vi "SmartSEM Remote API get float.vi"(8 "error in":errorcluster, 10 "lpszParam":string, 11 "ActiveX Container":refnum<k7>(container)) -> (0 "error out":errorcluster, 2 "vValue":sgl, 3 "reference out":refnum<k7>)   [LabVIEW 2018]
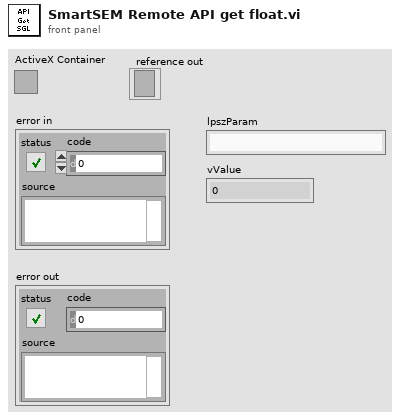
[diagram p1: front panel]
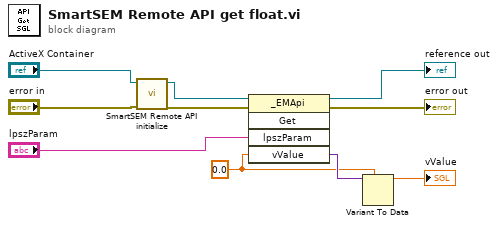
[diagram p0: block diagram]
diagram:
  w6 = sgl 0.0 ("vValue")
  n1 = call "SmartSEM Remote API initialize.vi"("error in"="error in", "ActiveX Container"="ActiveX Container") -> ("error out"=w1:errorcluster, "reference out"=w3:refnum<k7>)  [unwired: 8 in]
  n2 = invoke class="_EMApi" method="Get"(reference=w3, error in=w1, "lpszParam"="lpszParam", "vValue"=w6) -> (reference out=→"reference out":refnum<k7>, error out=→"error out":errorcluster, "vValue"=w7:variant)  [unwired: 1 in, 2 out]
  n3 = Variant To Data(type=w6, Variant=w7) -> (data=→"vValue":sgl)  [unwired: 1 in, 1 out]
